vi "test_ScanHeadDL090202.vi"() -> ()   [LabVIEW 2010, in "ScanHeadDL090202.lvclass"]
uses:
  ScanHeadDL090202.lvclass
  main/labview_source/type_definitions/enumerations/run_mode_enum.ctl
  main/labview_source/type_definitions/clusters/controls_refs.ctl
  Trajectory/TrajectoryDL090201FrameScan/TrajectoryDL090201FrameScan/TrajectoryDL090201FrameScan.lvclass
  common/classes/ErrorController/ErrorController/ErrorController.lvclass
  GenericScanHead/GenericScanHead/GenericScanHead.lvclass
  Trajectory/GenericTrajectory/GenericTrajectory/GenericTrajectory.lvclass
  GenericScanHead/GenericScanHead/trigger_enum.ctl
  common/classes/ErrorController/ErrorController/class_data.vi
  common/classes/GenericComponent/GenericComponent/GenericComponent.lvclass
panel:
  out "error loaded?":bool
  in  "create Trajectory button":bool
  in  "create ScanHead button":bool
  in  "mode":T1=enum."single sweep mode"
  in  "y ratio factor":dbl=1.0 caption="y"
  in  "x ratio factor":dbl=1.0 caption="x"
  in  "repetitions":i32=3
  in  "send trajectory":bool
  in  "repetition rate":dbl[unit]=10.0
  in  "y resolution":i32=256
  in  "x resolution":i32=256
  in  "stop":bool
  in  "scan start":bool
  # "Test DL090202ScanHead"
  # "The front panel of the ScanHead component will be loaded here..."
  # "Trajecotry settings"
  # "x:y ratio"
  # ":"
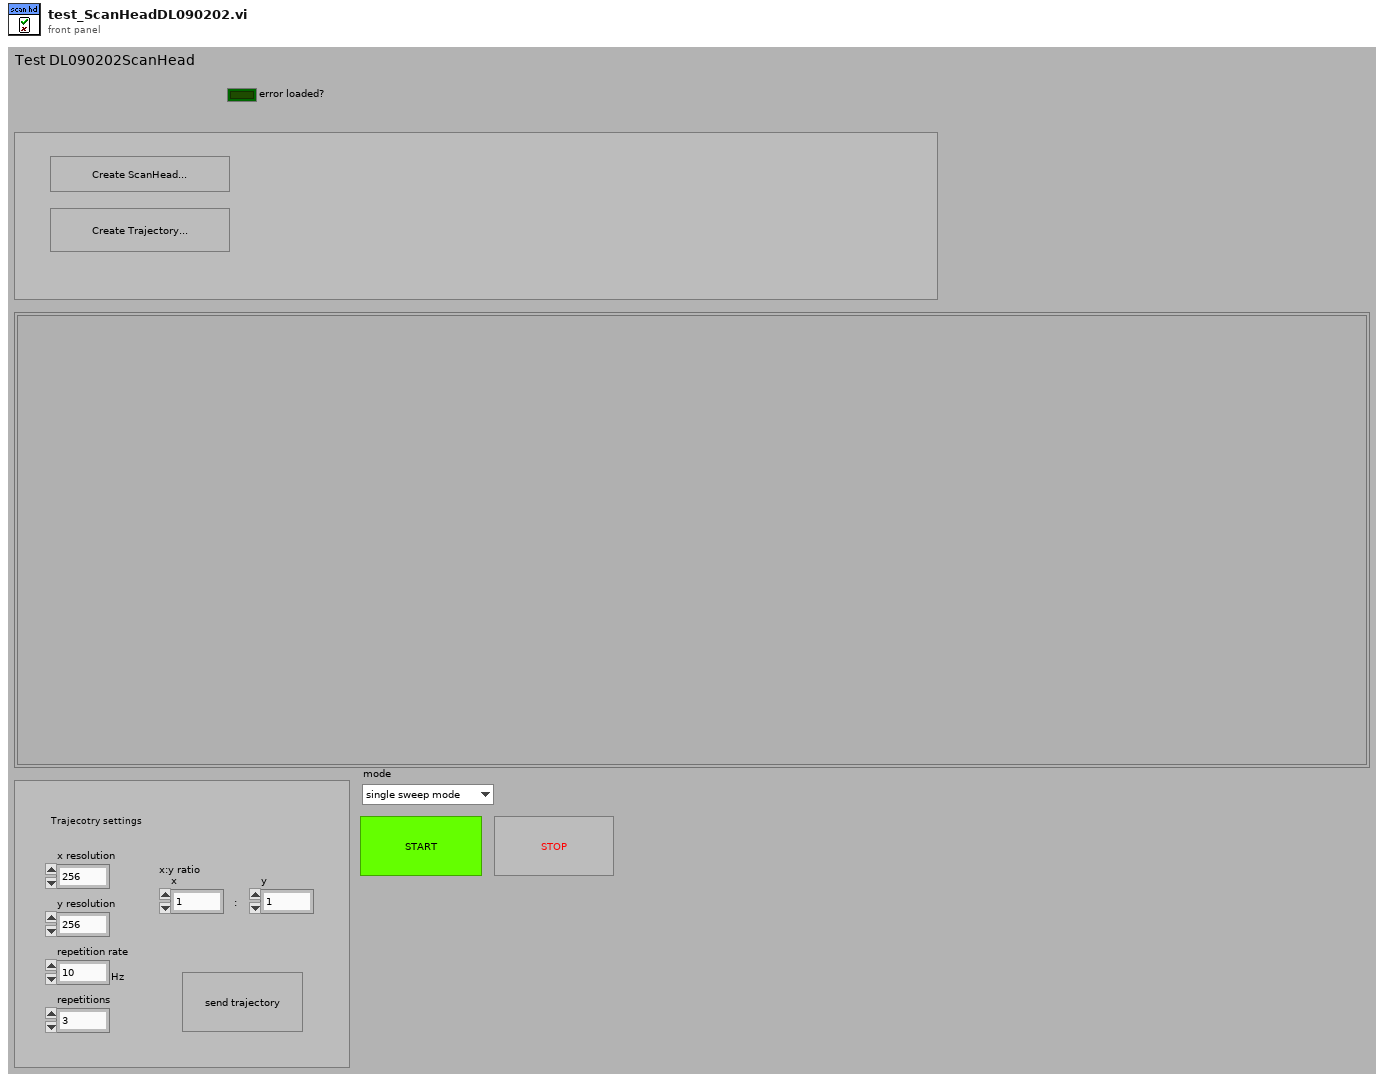
[diagram p1: front panel]
types:
  T1 = typedef "run_mode_enum.ctl" = enum16{"focus mode", "single sweep mode", "experiment mode"}
  T2 = typedef "controls_refs.ctl" = cluster{"buttons":cluster{"start_focus":refnum<vi>, "start_single_sweep":refnum<vi>, "start_experiment":refnum<vi>, "save":refnum<vi>, "exit":refnum<vi>}, "tabs":cluster{"main":refnum<vi>, "settings":refnum<vi>}, "subpanels":cluster{"imagingMode":refnum<vi>, "scanHead":refnum<vi>, "display":refnum<vi>, "experimentController":refnum<vi>, "instrument":refnum<vi>, "stage":refnum<vi>, "stimulator":refnum<vi>, "dataCollection":refnum<vi>, "analyser":refnum<vi>, "daq":refnum<vi>, "imageAssembler":refnum<vi>}, "drop-downs":cluster{"imagingMode":refnum<vi>, "experimentalController":refnum<vi>, "objective":refnum<vi>}, "status lights":cluster{"experimentController":refnum<vi>, "imagingMode":refnum<vi>, "scanHead":refnum<vi>, "daq":refnum<vi>, "imageAssembler":refnum<vi>, "dataCollection":refnum<vi>, "display":refnum<vi>, "analyser":refnum<vi>, "stage":refnum<vi>, "stimulator":refnum<vi>, "instrument":refnum<vi>}, "message":refnum<vi>, "stimulator enabled?":refnum<vi>, "saving":cluster{"data folder path":refnum<vi>, "file base name":refnum<vi>, "notebook":refnum<vi>}, "progress bar":refnum<vi>, "update icon":refnum<vi>, "title":refnum<vi>, "main vi":refnum<vi>, "user":refnum<vi>}
  T3 = typedef "GenericScanHead.lvclass/trigger_enum.ctl" = enum16{"NULL", "fetch trajectory", "generate trajectory", "change run mode", "update modifiers"}
  T4 = typedef "plugin_specification.ctl" = cluster{"class path":string, "configuration":string, "label":string, "settings name":string}
  T5 = typedef "XComponentSpecification.xctl/data.ctl" = cluster{"class path":string, "configuration":string, "label":string, "settings name":string}
  T6 = typedef "GenericToplevelComponent.lvclass/common_trigger_enum.ctl" = enum16{"NULL", "initialise", "terminate", "fetch command", "fetch data", "attach observer", "register as observer", "detach observer", "acknowledge", "start", "stop", "sweep started", "sweep finished", "experiment started", "experiment stopped"}
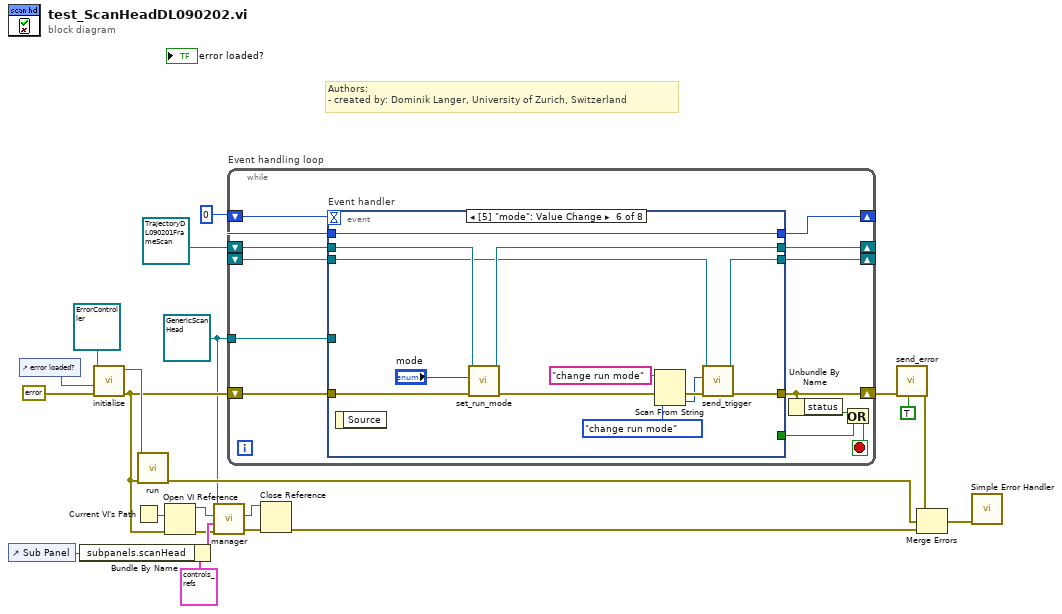
[diagram p0: block diagram]
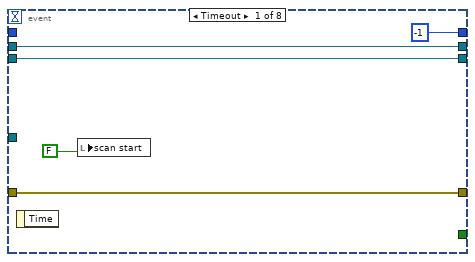
[diagram p2: hidden frame]
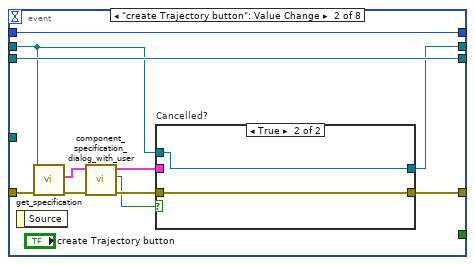
[diagram p3: hidden frame]
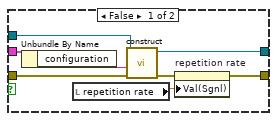
[diagram p4: hidden frame]
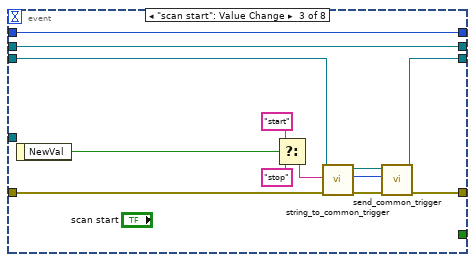
[diagram p5: hidden frame]
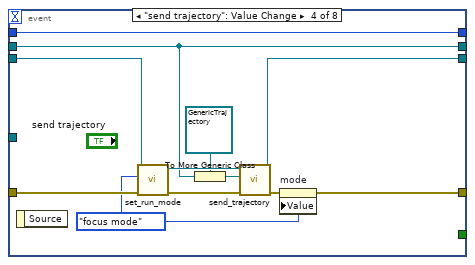
[diagram p6: hidden frame]
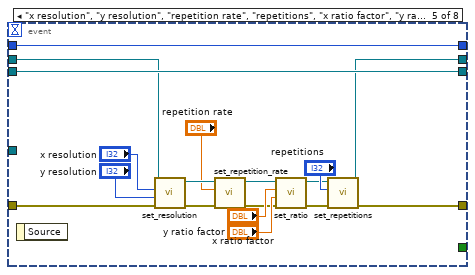
[diagram p7: hidden frame]
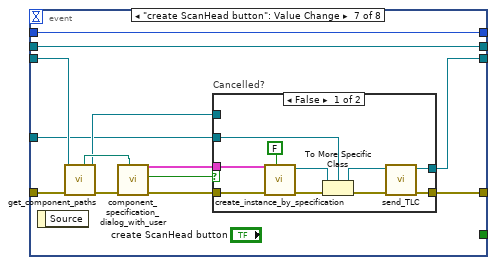
[diagram p8: hidden frame]
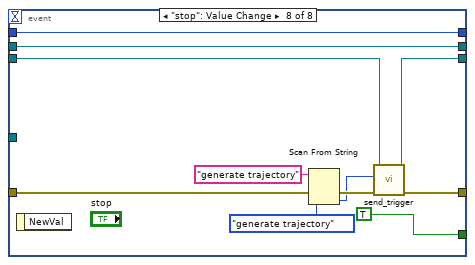
[diagram p10: hidden frame]
diagram:
  w2 = refnum<class "GenericScanHead.lvclass"> refnum ("GenericScanHead.lvclass")
  # "Authors: \n- created by: Dominik Langer, University of Zurich, Switzerland"
  n1 = control-ref of="Sub Panel"() -> (w20:refnum<vi>)
  n2 = control-ref of="error loaded?"() -> (w9:refnum<vi>)
  n3 = Bundle By Name(cluster=T2 {"buttons"={"start_focus"=refnum, "start_single_sweep"=refnum, "start_experiment"=refnum, "save"=refnum, "exit"=refnum}, "tabs"={"main"=refnum, "settings"=refnum}, "subpanels"={"imagingMode"=refnum, "scanHead"=refnum, "display"=refnum, "experimentController"=refnum, "instrument"=refnum, "stage"=refnum, "stimulator"=refnum, "dataCollection"=refnum, "analyser"=refnum, "daq"=refnum, "imageAssembler"=refnum}, "drop-downs"={"imagingMode"=refnum, "experimentalController"=refnum, "objective"=refnum}, "status lights"={"experimentController"=refnum, "imagingMode"=refnum, "scanHead"=refnum, "daq"=refnum, "imageAssembler"=refnum, "dataCollection"=refnum, "display"=refnum, "analyser"=refnum, "stage"=refnum, "stimulator"=refnum, "instrument"=refnum}, "message"=refnum, "stimulator enabled?"=refnum, "saving"={"data folder path"=refnum, "file base name"=refnum, "notebook"=refnum}, "progress bar"=refnum, "update icon"=refnum, "title"=refnum, "main vi"=refnum, "user"=refnum} ("control references"), "subpanels.scanHead"=w20) -> (w6:T2)
  n4 = call-dynamic "initialise.vi"("error in (no error)"=errorcluster {"status"=FALSE, "code"=0, "source"=""} ("error out"), "error boolean"=w9, "ErrorController in"=refnum<class "ErrorController.lvclass"> refnum ("ErrorController.lvclass")) -> ("error out"=w8:errorcluster, "ErrorController out"=w14:refnum<class "ErrorController.lvclass">)  [unwired: 7 in]
  n5 = Current VI's Path() -> (path=w17:path)
  n6 = call "run.vi"("error in (no error)"=w8, "ErrorController in"=w14) -> ("error out"=w13:errorcluster)  [unwired: 8 in, 1 out]
  n7 = Open VI Reference(vi path=w17, error in (no error)=w8) -> (vi reference=w5:refnum<vi>, error out=w4:errorcluster)  [unwired: 4 in]
  n8 = call-dynamic "manager.vi"("error in (no error)"=w4, "control references"=w6, "top-level VI ref in"=w5, "GenericToplevelComponent in"=w2) -> ("error out"=w3:errorcluster, "top-level VI ref out"=w1:refnum<vi>)  [unwired: 5 in, 1 out]
  n9 = while "Event handling loop" {
    shift-right: [w27] -> w12
    shift-left: w8 -> [w34]
    shift-right: [w32] -> _
    shift-left: 0 -> [w33]
    shift-right: [w28] -> _
    shift-left: _ -> [w31]
    shift-right: [w29] -> _
    shift-left: refnum<class "TrajectoryDL090201FrameScan.lvclass"> refnum ("TrajectoryDL090201FrameScan.lvclass") -> [w30]
    tunnel: w2 -> [w23]
    stop <- w24 stop-if-true
    n10 = event "Event handler" shown="[5] \"mode\": Value Change" {
      selector: _ -> [_ _ _ _ _ _ _ _]
      dyn-events: _ -> [_ _ _ _ _ _ _ _]
      timeout: w33 -> [_ _ _ _ _ _ _ _]
      tunnel: w34 -> [w35 w45 w66 w81 w100 w115 w124 w146]
      tunnel: [w35 w48 w67 w82 w102 w111 w128 w149] -> w27
      tunnel: [-1 w50 w73 w85 w103 w116 w129 w152] -> w32
      tunnel: w33 -> [_ w50 w73 w85 w103 w116 w129 w152]
      tunnel: [_ _ _ _ _ _ _ TRUE] -> w25
      tunnel: [w37 w49 w68 w84 w93 w109 w127 w147] -> w28
      tunnel: w31 -> [w37 w49 w63 w78 w93 w110 w125 w148]
      tunnel: w30 -> [w36 w46 w71 w74 w92 w113 w126 w150]
      tunnel: [w36 w47 w71 w74 w91 w112 w126 w150] -> w29
      tunnel: w23 -> [_ _ _ _ _ _ w117 _]
      event Timeout {
        n11 = event-data() -> ()  [unwired: 2 out]
        n12 = local write "scan start"(FALSE) -> ()
      }
      event "create Trajectory button": Value Change {
        n13 = event-data() -> ()  [unwired: 2 out]
        n14 = call-dynamic "get_specification.vi"("error in (no error)"=w45, "GenericPlugin in"=w46) -> ("error out"=w43:errorcluster, "component specification"=w44:T4)  [unwired: 6 in, 2 out]
        n15 = call "component_specification_dialog_with_user.vi"("error in (no error)"=w43, "component specification in"=w44) -> ("error out"=w42:errorcluster, "cancelled?"=w40:bool, "component specification out"=w41:T5)  [unwired: 7 in]
        n16 = case "Cancelled?" shown="True" w40 {
          tunnel: [w56 w60] -> w48
          tunnel: [w55 w59] -> w47
          tunnel: w46 -> [w54 w59]
          tunnel: w42 -> [w53 w60]
          tunnel: w41 -> [w52 _]
          frame False {
            n17 = Unbundle By Name(w52) -> ("configuration"=w51:string)
            n18 = local read "repetition rate"() -> (w58:dbl[unit])
            n19 = call-dynamic "construct.vi"("error in (no error)"=w53, "configuration name"=w51, "GenericPlugin in"=w54) -> ("error out"=w57:errorcluster, "GenericPlugin out"=w55:refnum<class "TrajectoryDL090201FrameScan.lvclass">)  [unwired: 1 in, 6 out]
            n20 = property on="repetition rate" class="DigNum (strict)"(error in=w57, "Val(Sgnl)"=w58) -> (error out=w56:errorcluster)  [unwired: 1 in, 1 out]
          }
          frame True {
          }
        }
      }
      event "scan start": Value Change {
        n21 = event-data() -> ("NewVal"=w72:bool)  [unwired: 1 out]
        n22 = Select(t="start", s=w72, f="stop") -> (s? t:f=w69:string)
        n23 = call-dynamic "string_to_common_trigger.vi"("error in (no error)"=w66, "trigger string"=w69, "GenericToplevelComponent in"=w63) -> ("error out"=w65:errorcluster, "trigger"=w64:T6, "GenericToplevelComponent out"=w62:refnum<class "GenericScanHead.lvclass">)  [unwired: 6 in]
        n24 = call-dynamic "send_common_trigger.vi"("error in (no error)"=w65, "trigger"=w64, "GenericToplevelComponent in"=w62) -> ("error out"=w67:errorcluster, "GenericToplevelComponent out"=w68:refnum<class "GenericScanHead.lvclass">)  [unwired: 6 in, 1 out]
      }
      event "send trajectory": Value Change {
        w79 = run_mode_enum."focus mode" ("mode")
        n25 = event-data() -> ()  [unwired: 2 out]
        n26 = call-dynamic "set_run_mode.vi"("error in (no error)"=w81, "run mode"=w79, "GenericPlugin in"=w78) -> ("error out"=w80:errorcluster, "GenericPlugin out"=w77:refnum<class "GenericScanHead.lvclass">)  [unwired: 7 out]
        n27 = To More Generic Class(target class=refnum<class "GenericTrajectory.lvclass"> refnum ("trajectory"), reference=w74) -> (generic class reference=w75:refnum<class "GenericTrajectory.lvclass">)
        n28 = call-dynamic "send_trajectory.vi"("error in (no error)"=w80, "trajectory"=w75, "GenericScanHead in"=w77) -> ("error out"=w83:errorcluster, "GenericScanHead out"=w84:refnum<class "GenericScanHead.lvclass">)  [unwired: 7 out]
        n29 = property on="mode" class="Enum (strict)"(error in=w83, "Value"=w79) -> (error out=w82:errorcluster)  [unwired: 1 in, 1 out]
      }
      event "x resolution", "y resolution", "repetition rate", "repetitions", "x ratio factor", "y ratio factor": Value Change {
        n30 = event-data() -> ()  [unwired: 2 out]
        n31 = call-dynamic "set_resolution.vi"("error in (no error)"=w100, "y"="y resolution", "x"="x resolution", "TrajectoryDL090201FrameScan in"=w92) -> ("error out"=w90:errorcluster, "TrajectoryDL090201FrameScan out"=w87:refnum<class "TrajectoryDL090201FrameScan.lvclass">)  [unwired: 6 out]
        n32 = call-dynamic "set_repetition_rate.vi"("error in (no error)"=w90, "repetition rate"="repetition rate", "GenericTrajectory in"=w87) -> ("error out"=w89:errorcluster, "GenericTrajectory out"=w88:refnum<class "TrajectoryDL090201FrameScan.lvclass">)  [unwired: 7 in]
        n33 = call-dynamic "set_ratio.vi"("error in (no error)"=w89, "y"="y ratio factor", "x"="x ratio factor", "TrajectoryDL090201FrameScan in"=w88) -> ("error out"=w97:errorcluster, "TrajectoryDL090201FrameScan out"=w96:refnum<class "TrajectoryDL090201FrameScan.lvclass">)  [unwired: 6 out]
        n34 = call-dynamic "set_repetitions.vi"("error in (no error)"=w97, "repetitions"="repetitions", "GenericTrajectory in"=w96) -> ("error out"=w102:errorcluster, "GenericTrajectory out"=w91:refnum<class "TrajectoryDL090201FrameScan.lvclass">)  [unwired: 7 out]
      }
      event Value Change {
        n35 = event-data() -> ()  [unwired: 2 out]
        n36 = call-dynamic "set_run_mode.vi"("error in (no error)"=w115, "run mode"="mode", "GenericPlugin in"=w113) -> ("error out"=w108:errorcluster, "GenericPlugin out"=w112:refnum<class "TrajectoryDL090201FrameScan.lvclass">)  [unwired: 7 out]
        n37 = Scan From String(input string="change run mode", error in=w108, default 1=trigger_enum."change run mode" ("trigger")) -> (error out=w107:errorcluster, output 1=w106:T3)  [unwired: 2 in, 2 out]
        n38 = call-dynamic "send_trigger.vi"("error in (no error)"=w107, "trigger"=w106, "GenericScanHead in"=w110) -> ("error out"=w111:errorcluster, "GenericScanHead out"=w109:refnum<class "GenericScanHead.lvclass">)  [unwired: 7 out]
      }
      event "create ScanHead button": Value Change {
        n39 = event-data() -> ()  [unwired: 2 out]
        n40 = call-dynamic "get_component_paths.vi"("error in (no error)"=w124, "GenericComponent in"=w125) -> ("error out"=w122:errorcluster, "GenericComponent out"=w119:refnum<class "GenericScanHead.lvclass">, "component type directory"=w120:path)  [unwired: 4 in, 3 out]
        n41 = call "component_specification_dialog_with_user.vi"("start path"=w120, "error in (no error)"=w122) -> ("error out"=w121:errorcluster, "cancelled?"=w123:bool, "component specification out"=w118:T5)  [unwired: 7 in]
        n42 = case "Cancelled?" shown="False" w123 {
          tunnel: [w139 w141] -> w128
          tunnel: [w138 w140] -> w127
          tunnel: w121 -> [w132 w141]
          tunnel: w119 -> [_ w140]
          tunnel: w118 -> [w131 _]
          tunnel: w117 -> [w130 _]
          frame False {
            n43 = call "create_instance_by_specification.vi"("call constructor?"=FALSE, "error in (no error)"=w132, "component specification"=w131) -> ("error out"=w137:errorcluster, "GenericPlugin out"=w134:refnum<class "GenericComponent.lvclass">)  [unwired: 6 in, 1 out]
            n44 = To More Specific Class(target class=w130, reference=w134, error in=w137) -> (specific class reference=w135:refnum<class "GenericScanHead.lvclass">, error out=w136:errorcluster)
            n45 = call-dynamic "send_TLC.vi"("error in (no error)"=w136, "GenericToplevelComponent in"=w135) -> ("error out"=w139:errorcluster, "GenericToplevelComponent out"=w138:refnum<class "GenericScanHead.lvclass">)  [unwired: 8 in]
          }
          frame True {
          }
        }
      }
      event "stop": Value Change {
        n46 = event-data() -> ()  [unwired: 2 out]
        n47 = Scan From String(input string="generate trajectory", error in=w146, default 1=trigger_enum."generate trajectory" ("trigger")) -> (error out=w145:errorcluster, output 1=w143:T3)  [unwired: 2 in, 2 out]
        n48 = call-dynamic "send_trigger.vi"("error in (no error)"=w145, "trigger"=w143, "GenericScanHead in"=w148) -> ("error out"=w149:errorcluster, "GenericScanHead out"=w147:refnum<class "GenericScanHead.lvclass">)  [unwired: 7 out]
      }
    }
    n49 = Unbundle By Name(w27) -> ("status"=w26:bool)
    n50 = Or(x=w26, y=w25) -> (x .or. y?=w24:bool)
  }
  n51 = Close Reference(reference=w1, error in (no error)=w3) -> (error out=w18:errorcluster)
  n52 = call "send_error.vi"("last error? (F)"=TRUE, "error in (no error)"=w12) -> ("error out"=w11:errorcluster)  [unwired: 9 in]
  n53 = Merge Errors(w11, w13, w18) -> (w21:errorcluster)
  n54 = call <vilib>:"Simple Error Handler.vi"("error in (no error)"=w21) -> ()  [unwired: 1 in, 8 out]
